vi "FIR Filter (DBL).vi"(2 "init/cont (init:F)":bool, 3 "FIR Coefficients":dbl[](array[numeric]), 5 "X":dbl[](array[numeric])) -> (0 "error":i32, 1 "Filtered X":dbl[](array[numeric]))   [LabVIEW 2017, in "NI_AALBase.lvlib"]
doc: "Filters the input sequence<B> X</B> using the direct-form FIR filter specified by <B>FIR Coefficients</B>. Wire data to the <B>X</B> input to determine the polymorphic instance to use or manually select the instance."
uses:
  NI_AALBase.lvlib
  lvanlys.dll
panel:
  # "FIR Filter"
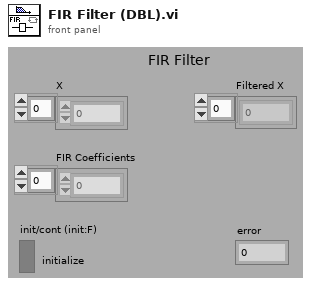
[diagram p1: front panel]
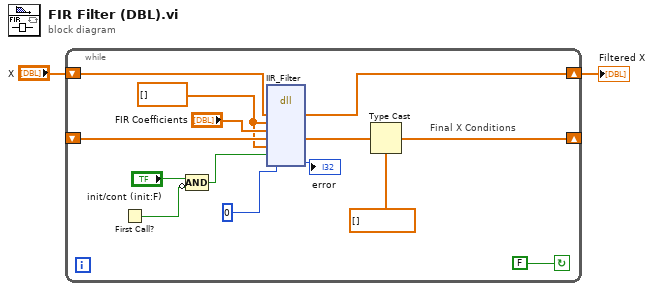
[diagram p0: block diagram]
diagram:
  n1 = while {
    shift-left: _ -> [w11]
    shift-right: [w16] -> _
    shift-right: [w4] -> w1
    shift-left: "X" -> [w5]
    stop <- FALSE continue-if-true
    w3 = dbl[] [] ("Reverse Coefficients")
    # "Final X Conditions"
    n2 = First Call?() -> (First Call?: T/F=w7:bool)
    n3 = Compound Arithmetic op=AND("init/cont (init:F)", invert w7) -> (w6:bool)
    n4 = dll-call lib="C:/Program Files/National Instruments/LabVIEW 2017/resource/lvanlys.*" fn="IIR_Filter"("X"=w5, "Reverse Coefficients"=w3, "FIR Coefficients"="FIR Coefficients", "type for the shift register"=w11, "Reverse Coefficients"=w3, "output param"=w6, "output param"=0) -> ("X"=w4:dbl[], "type for the shift register"=w10:dbl[], "output param"=→"error":i32)  [unwired: 8 in, 2 out]
    n5 = Type Cast(type=dbl[] [] ("type for the shift register"), x=w10) -> (*(type *) &x=w16:dbl[])
  }
  "Filtered X" <- w1
